vi "Parse I2C Messages.vi"(7 "Timestamp ID":T1, 8 "error in (no error)":errorcluster, 11 "User Timestamps":u64[](array[numeric])) -> (0 "error out":errorcluster, 2 "Count":i32, 3 "I2C Messages":string[][](array[string]))   [LabVIEW 2025, in "I2C Bus Monitor.lvclass"]
uses:
  <instrlib>/FlexRIO/CSI-2/v2/FPGA/Types/Timestamp ID.ctl
  <instrlib>/FlexRIO/CSI-2/v2/FPGA/Types/Raw Timestamp.ctl
  <instrlib>/FlexRIO/CSI-2/v2/Host/subVIs/Convert Raw Timestamp to User Timestamp.vi
  I2C Bus Monitor.lvclass
  I2C Bus Monitor.lvclass/I2C Bus Monitor.ctl
  <instrlib>/FlexRIO/CSI-2/v2/FPGA/NI CSI-2 API FPGA v2.lvlib
  <instrlib>/FlexRIO/CSI-2/v2/Host/NI CSI-2 API Host v2.lvlib
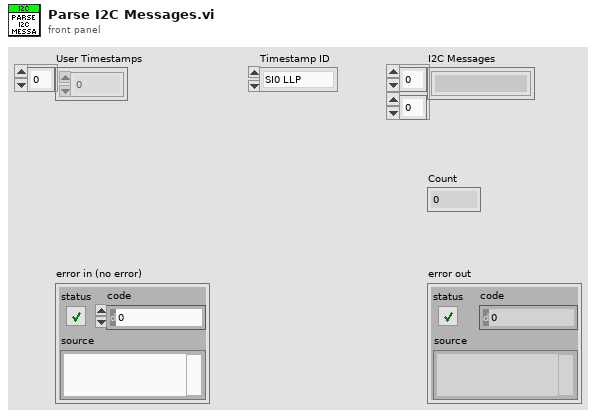
[diagram p1: front panel]
types:
  T1 = typedef "NI CSI-2 API FPGA v2.lvlib/Timestamp ID.ctl" = enum8{"SI0 LLP", "SI1 LLP", "SI2 LLP", "SI3 LLP", "SI4 LLP", "SI5 LLP", "SI6 LLP", "SI7 LLP", "SO0 LLP", "SO1 LLP", "SO2 LLP", "SO3 LLP", "SO4 LLP", "SO5 LLP", "SO6 LLP", "SO7 LLP", "Ser0 GPIO Bank", "Ser1 GPIO Bank", "Ser2 GPIO Bank", "Ser3 GPIO Bank", "Ser4 GPIO Bank", "Ser5 GPIO Bank", "Ser6 GPIO Bank", "Ser7 GPIO Bank", "Des0 GPIO Bank", "Des1 GPIO Bank", "Des2 GPIO Bank", "Des3 GPIO Bank", "Des4 GPIO Bank", "Des5 GPIO Bank", "Des6 GPIO Bank", "Des7 GPIO Bank", "User0", "User1", "User2", "User3", "User4", "User5", "User6", "User7", "User8", "User9", "User10", "User11", "User12", "User13", "User14", "User15", "User16", "User17", "User18", "User19", "User20", "User21", "User22", "User23", "User24", "User25", "User26", "User27", "User28", "User29", "User30", "User31"}
  T2 = typedef "NI CSI-2 API FPGA v2.lvlib/Raw Timestamp.ctl" = cluster{"timestamp":u64, "valid":bool}
  T3 = typedef "NI CSI-2 API FPGA v2.lvlib/User Timestamp.ctl" = cluster{"valid":bool, "user data":fxp<+,58,58>, "id":T1}
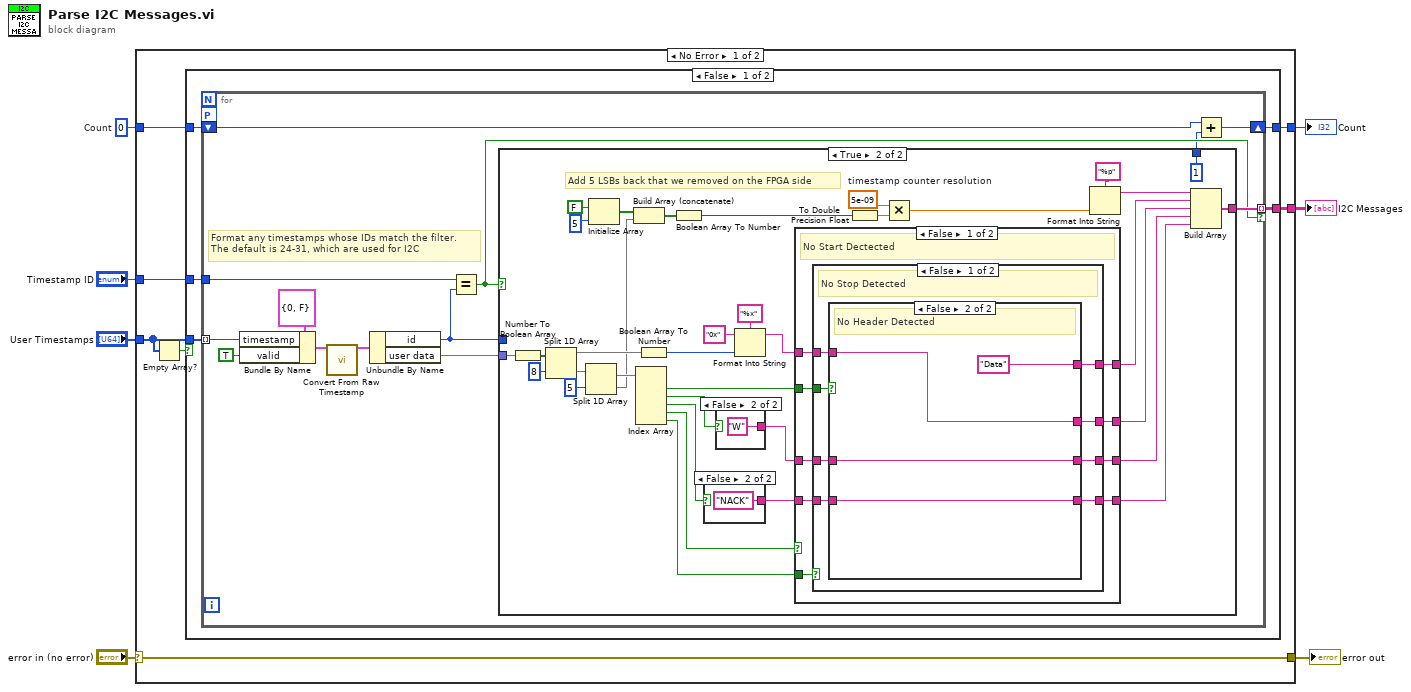
[diagram p0: block diagram]
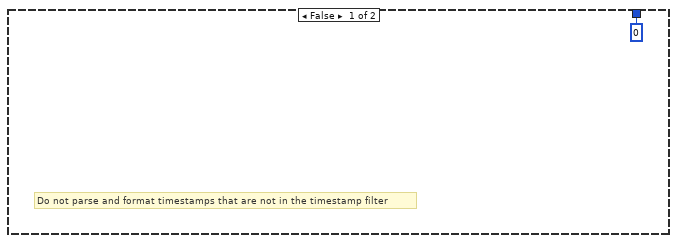
[diagram p2: hidden frame]
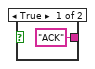
[diagram p3: hidden frame]
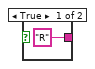
[diagram p4: hidden frame]
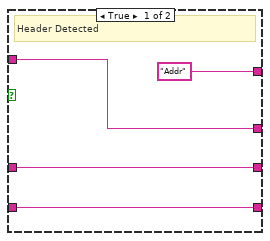
[diagram p5: hidden frame]
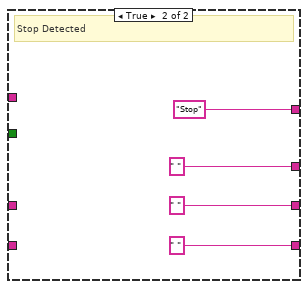
[diagram p6: hidden frame]
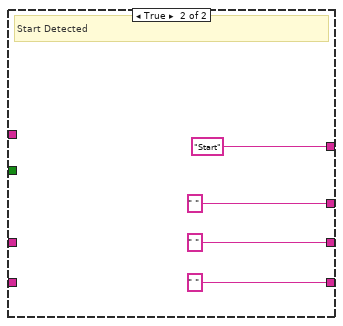
[diagram p7: hidden frame]
diagram:
  w5 = 0  # Count
  n1 = case shown="No Error" "error in (no error)" {
    selector: "error in (no error)" -> [w10 w106]
    tunnel: "User Timestamps" -> [w9 _]
    tunnel: "Timestamp ID" -> [w14 _]
    tunnel: w5 -> [w13 _]
    tunnel: [w12 _] -> w4
    tunnel: [w11 _] -> w3
    tunnel: [w10 w106] -> w1
    frame No Error {
      n2 = Empty Array?(array=w9) -> (empty?=w8:bool)
      n3 = case shown="False" w8 {
        tunnel: w14 -> [w19 _]
        tunnel: w13 -> [w18 _]
        tunnel: [w17 _] -> w12
        tunnel: [w16 _] -> w11
        tunnel: w9 -> [w15 _]
        frame False {
          n4 = for {
            tunnel: [w32] -> w17 mode=indexing if=w29
            workers-P: _ -> [_]
            shift-right: [w27] -> w16
            shift-left: w18 -> [w26]
            tunnel: w19 -> [w25]
            tunnel: w15 -> [w21] mode=indexing
            # "Format any timestamps whose IDs match the filter.\nThe default is 24-31, which are used for I2C"
            n5 = Bundle By Name(cluster=T2 {"timestamp"=0, "valid"=FALSE} ("raw timestamp"), "timestamp"=w21, "valid"=TRUE) -> (w23:T2)
            n6 = call-poly <instrlib>:"Convert From Raw Timestamp.vi"("raw timestamp"=w23) -> ("user timestamp"=w20:T3)  [unwired: 14 in]
            n7 = Unbundle By Name(w20) -> ("id"=w30:T1, "user data"=w31:fxp<+,58,58>)
            n8 = Equal?(x=w25, y=w30) -> (x = y?=w29:bool)
            n9 = case shown="True" w29 {
              tunnel: [_ w67] -> w32
              tunnel: w31 -> [_ w62]
              tunnel: w30 -> [_ _]
              tunnel: [0 ("x") 1 ("x")] -> w28
              frame False {
                # "Do not parse and format timestamps that are not in the timestamp filter"
              }
              frame True {
                w65 = 5e-09  # timestamp counter resolution
                # "Add 5 LSBs back that we removed on the FPGA side"
                n10 = Number To Boolean Array(number=w62) -> (Boolean array=w61:bool[])
                n11 = Split 1D Array(array=w61, index=8) -> (first subarray=w56:bool[], second subarray=w59:bool[])
                n12 = Split 1D Array(array=w59, index=5) -> (first subarray=w57:bool[], second subarray=w34:bool[])
                n13 = Initialize Array(FALSE, 5 ("dimension size")) -> (w53:bool[])
                n14 = Build Array (concatenate)(w53, w34) -> (w52:bool[])
                n15 = Index Array(array=w57) -> (element #1=w48:bool, element #2=w47:bool, element #3=w44:bool, element #4=w50:bool, element #5=w49:bool)  [unwired: 5 in]
                n16 = Boolean Array To Number(Boolean array=w56) -> (number=w38:u32)
                n17 = Boolean Array To Number(Boolean array=w52) -> (number=w51:u64)
                n18 = case shown="False" w44 {
                  tunnel: ["ACK" "NACK"] -> w45
                  frame True {
                  }
                  frame False {
                  }
                }
                n19 = case shown="False" w47 {
                  tunnel: ["R" "W"] -> w46
                  frame True {
                  }
                  frame False {
                  }
                }
                n20 = Format Into String(format string="%x", initial string="0x", w38) -> (resulting string=w37:string)  [unwired: 1 in, 1 out]
                n21 = case shown="False" w50 {
                  tunnel: w49 -> [w81 _]
                  tunnel: w48 -> [w80 _]
                  tunnel: w46 -> [w79 _]
                  tunnel: w45 -> [w78 _]
                  tunnel: w37 -> [w77 _]
                  tunnel: [w76 "Start"] -> w43
                  tunnel: [w75 " "] -> w36
                  tunnel: [w74 " "] -> w42
                  tunnel: [w73 " "] -> w41
                  frame False {
                    # "No Start Dectected"
                    n22 = case shown="False" w81 {
                      tunnel: w80 -> [w89 _]
                      tunnel: w79 -> [w88 _]
                      tunnel: w78 -> [w87 _]
                      tunnel: w77 -> [w86 _]
                      tunnel: [w85 "Stop"] -> w76
                      tunnel: [w84 " "] -> w75
                      tunnel: [w83 " "] -> w74
                      tunnel: [w82 " "] -> w73
                      frame False {
                        # "No Stop Detected"
                        n23 = case shown="False" w89 {
                          tunnel: w88 -> [w91 w95]
                          tunnel: w87 -> [w90 w94]
                          tunnel: w86 -> [w92 w96]
                          tunnel: ["Addr" "Data"] -> w85
                          tunnel: [w92 w96] -> w84
                          tunnel: [w91 w95] -> w83
                          tunnel: [w90 w94] -> w82
                          frame True {
                            # "Header Detected"
                          }
                          frame False {
                            # "No Header Detected"
                          }
                        }
                      }
                      frame True {
                        # "Stop Detected"
                      }
                    }
                  }
                  frame True {
                    # "Start Detected"
                  }
                }
                n24 = To Double Precision Float(number=w51) -> (double precision float=w64:dbl)
                n25 = Multiply(x=w65, y=w64) -> (x*y=w66:dbl)
                n26 = Format Into String(format string="%p", w66) -> (resulting string=w68:string)  [unwired: 2 in, 1 out]
                n27 = Build Array(w68, w43, w36, w42, w41) -> (w67:string[])
              }
            }
            n28 = Add(x=w26, y=w28) -> (x+y=w27:i32)
          }
        }
        frame True {
        }
      }
    }
    frame Error {
    }
  }
  "I2C Messages" <- w4
  "Count" <- w3
  "error out" <- w1
